vi "Make Plot Labels.vi"(0 "Plot Size":i32=-10, 1 "Column Headings":string[](array[string]), 2 "Display?":bool[](array[boolean])=[FALSE, FALSE, FALSE, FALSE, FALSE, FALSE, FALSE, FALSE, FALSE, FALSE, FALSE, FALSE, FALSE, FALSE, FALSE, FALSE, FALSE], 3 "# of columns":i32=-10, 4 "X-axis":i32=-10) -> (5 "Plot Names":string[](array[string]))   [LabVIEW 2020]
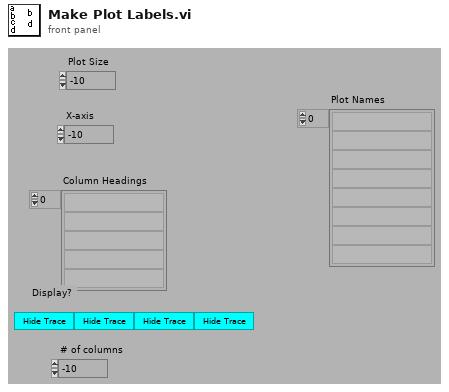
[diagram p1: front panel]
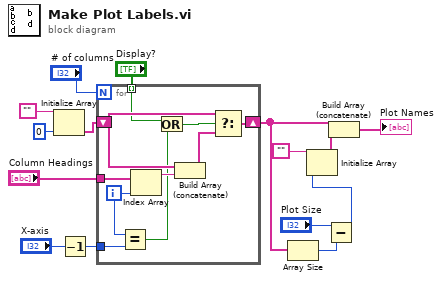
[diagram p0: block diagram]
diagram:
  n1 = Initialize Array("" ("f"), 0) -> (w15:string[])
  n2 = Decrement(x="X-axis") -> (x-1=w1:i32)
  n3 = for {
    N: "# of columns" -> [_]
    shift-right: [w24] -> w4
    shift-left: w15 -> [w23]
    tunnel: "Column Headings" -> [w25]
    tunnel: "Display?" -> [w20] mode=indexing
    tunnel: w1 -> [w19]
    i -> [w18]
    n4 = Equal?(x=w18, y=w19) -> (x = y?=w16:bool)
    n5 = Index Array(array=w25, index=w18) -> (element=w21:string)
    n6 = Or(x=w20, y=w16) -> (x .or. y?=w17:bool)
    n7 = Build Array (concatenate)(w23, w21) -> (w22:string[])
    n8 = Select(t=w23, s=w17, f=w22) -> (s? t:f=w24:string[])
  }
  n9 = Array Size(array=w4) -> (size(s)=w5:i32)
  n10 = Subtract(x="Plot Size", y=w5) -> (x-y=w3:i32)
  n11 = Initialize Array("" ("f"), w3) -> (w7:string[])
  n12 = Build Array (concatenate)(w4, w7) -> (→"Plot Names":string[])
